vi "Test Add.vi"(11 "Test Case In":refnum<class "Vector 2D Tests.lvclass">) -> (0 "error out":errorcluster, 3 "Test Case Out":refnum<class "Vector 2D Tests.lvclass">)   [LabVIEW 2021, in "Vector 2D Tests.lvclass"]
uses:
  Vector 2D Tests.lvclass
  4993e8ee-a06a-463a-9684-69129f64d5ce.vi
  Re-use Libraries/Vector 2D/Vector 2D.lvclass
  <vilib>/Astemes/LUnit/Test Case.lvclass
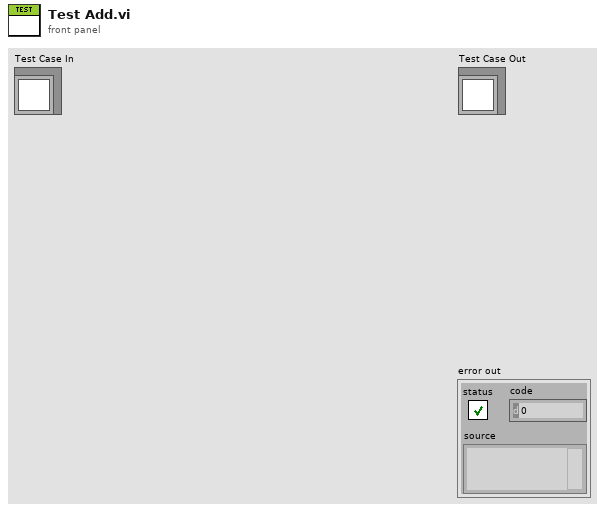
[diagram p1: front panel]
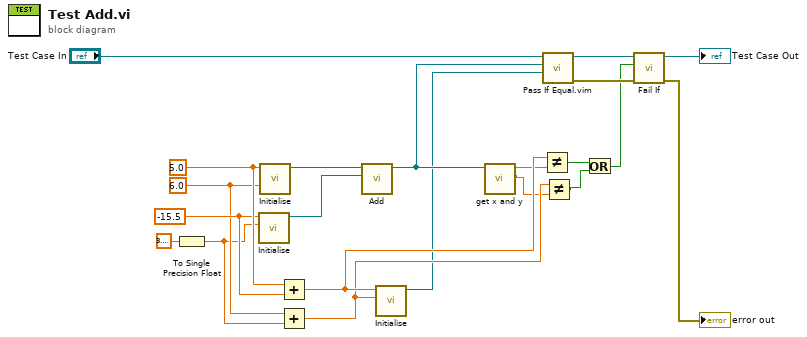
[diagram p0: block diagram]
diagram:
  w17 = sgl -15.5 ("x")
  w16 = sgl 6.0 ("y")
  w18 = sgl 5.0 ("x")
  n1 = To Single Precision Float(number=3.141592653589793) -> (single precision float=w15:sgl)
  n2 = call "Initialise.vi"("y"=w15, "x"=w17) -> ("Vector 2D out"=w14:refnum<class "Vector 2D.lvclass">)  [unwired: 9 in]
  n3 = call "Initialise.vi"("y"=w16, "x"=w18) -> ("Vector 2D out"=w20:refnum<class "Vector 2D.lvclass">)  [unwired: 9 in]
  n4 = Add(x=w18, y=w17) -> (x+y=w10:sgl)
  n5 = Add(x=w16, y=w15) -> (x+y=w8:sgl)
  n6 = call "Add.vi"("B"=w14, "A"=w20) -> ("A+B"=w11:refnum<class "Vector 2D.lvclass">)  [unwired: 9 in]
  n7 = call "Initialise.vi"("y"=w8, "x"=w10) -> ("Vector 2D out"=w1:refnum<class "Vector 2D.lvclass">)  [unwired: 9 in]
  n8 = call "get x and y.vi"("Vector 2D in"=w11) -> ("y"=w7:sgl, "x"=w9:sgl)  [unwired: 9 in]
  n9 = Not Equal?(x=w10, y=w9) -> (x != y?=w5:bool)
  n10 = call "Pass If Equal.vim"("Actual"=w1, "Expected"=w11, "LUnit Test Case In"="Test Case In") -> ("error out"=w6:errorcluster, "LUnit Test Case Out"=w13:refnum<class "Vector 2D Tests.lvclass">)  [unwired: 7 in]
  n11 = Not Equal?(x=w8, y=w7) -> (x != y?=w4:bool)
  n12 = Or(x=w5, y=w4) -> (x .or. y?=w3:bool)
  n13 = call <vilib>:"Fail If.vi"("error in (no error)"=w6, "Fail?"=w3, "LUnit Test Case In"=w13) -> ("error out"=→"error out":errorcluster, "LUnit Test Case Out"=→"Test Case Out":refnum<class "Vector 2D Tests.lvclass">)  [unwired: 7 in]
